vi "Data_GetEventReference.vi"(8 "error in (no error)":errorcluster, 11 "data":variant) -> (0 "error out":errorcluster, 1 "data group":string, 2 "event reference":T1, 3 "data out":variant, 5 "trend points only":bool, 7 "extra large file":bool)   [LabVIEW 2017, in "FileManager.lvlib"]
uses:
  <vilib>/addons/InsightCM/Devices/Shared/Common/FileManager/FileManager.lvlib
  <vilib>/addons/InsightCM/Devices/Shared/Common/DataEvent/controls/EventReference.ctl
  <vilib>/addons/InsightCM/Devices/Shared/Common/DataEvent/controls/Event.ctl
  <vilib>/addons/InsightCM/MessageBus/Base/controls/DataEvent.ctl
  <vilib>/addons/InsightCM/MessageBus/Base/controls/KeyValuePair.ctl
  <vilib>/addons/InsightCM/Devices/Shared/Common/DataEvent/controls/DataSet.ctl
  <vilib>/addons/InsightCM/MessageBus/Base/controls/DataSetMetadata.ctl
  <vilib>/addons/InsightCM/MessageBus/Base/controls/TrendPoint.ctl
  <vilib>/addons/InsightCM/MessageBus/Base/controls/TrendAlarmUpdate.ctl
  <vilib>/addons/InsightCM/MessageBus/Base/controls/TrendAlarmTransition.ctl
  <vilib>/addons/InsightCM/Devices/Shared/Common/FileManager/controls/DataPropertyNames.ctl
  <vilib>/addons/InsightCM/Devices/Shared/Common/DataEvent/DataEvent.lvlib
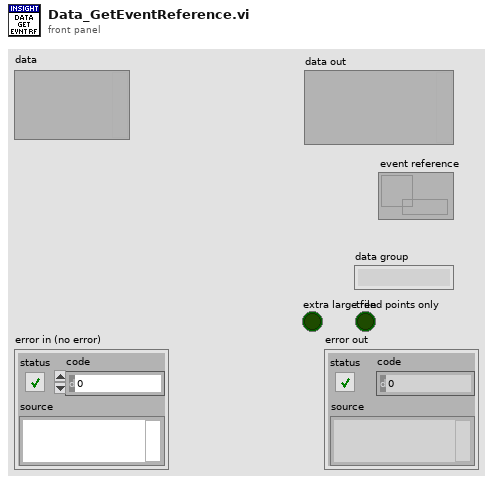
[diagram p1: front panel]
types:
  T1 = typedef "DataEvent.lvlib/EventReference.ctl" = refnum<data-value>
  T2 = typedef "DataPropertyNames.ctl" = enum16{"Type", "EventRef", "FilePath", "DataGroup", "AcquisitionTimestamp", "StreamId", "StreamBlock", "TrendPointsOnly", "ExtraLargeFile"}
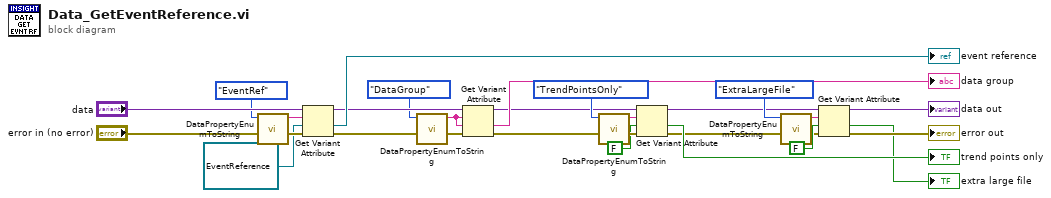
[diagram p0: block diagram]
diagram:
  n1 = call <vilib>:"DataPropertyEnumToString.vi"("property"=DataPropertyNames."EventRef" ("Names")) -> ("string"=w17:string)  [unwired: 10 in]
  n2 = Get Variant Attribute(Variant="data", name=w17, default value (empty Variant)=T1 refnum ("event reference"), error in="error in (no error)") -> (duplicate Variant=w21:variant, value=→"event reference":T1, error out=w20:errorcluster)  [unwired: 1 out]
  n3 = call <vilib>:"DataPropertyEnumToString.vi"("property"=DataPropertyNames."DataGroup" ("Names")) -> ("string"=w15:string)  [unwired: 10 in]
  n4 = Get Variant Attribute(Variant=w21, name=w15, default value (empty Variant)=w15, error in=w20) -> (duplicate Variant=w11:variant, value=→"data group":string, error out=w12:errorcluster)  [unwired: 1 out]
  n5 = call <vilib>:"DataPropertyEnumToString.vi"("property"=DataPropertyNames."TrendPointsOnly" ("Names")) -> ("string"=w14:string)  [unwired: 10 in]
  n6 = Get Variant Attribute(Variant=w11, name=w14, default value (empty Variant)=FALSE, error in=w12) -> (duplicate Variant=w5:variant, value=→"trend points only":bool, error out=w4:errorcluster)  [unwired: 1 out]
  n7 = call <vilib>:"DataPropertyEnumToString.vi"("property"=DataPropertyNames."ExtraLargeFile" ("Names")) -> ("string"=w6:string)  [unwired: 10 in]
  n8 = Get Variant Attribute(Variant=w5, name=w6, default value (empty Variant)=FALSE, error in=w4) -> (duplicate Variant=→"data out":variant, value=→"extra large file":bool, error out=→"error out":errorcluster)  [unwired: 1 out]
